vi "Default Settings.vi"(8 "error in (no error)":errorcluster, 11 "6 inch CAD Dispense in":refnum<class "6 inch CAD Dispense.lvclass">) -> (0 "error out":errorcluster, 3 "6 inch CAD Dispense out":refnum<class "6 inch CAD Dispense.lvclass">)   [LabVIEW 2020, in "6 inch CAD Dispense.lvclass"]
uses:
  6 inch CAD Dispense.lvclass
  Dispense.lvclass
  CAD Dispense.lvclass
  C:/Users/hep/Documents/CMU gantry/Classes/Routine/Dispense/CAD Dispense/CAD Dispense.lvclass
  C:/Users/hep/Documents/CMU gantry/Classes/Routine/Dispense/CAD Dispense/6 inch CAD Dispense.lvclass
  C:/Users/hep/Documents/CMU gantry/Classes/Routine/Routine.lvclass
  C:/Program Files/National Instruments/LabVIEW 2020/vi.lib/ActorFramework/Actor/Actor.lvclass
  C:/Users/hep/Documents/CMU gantry/Classes/Routine/Dispense/Dispense.lvclass
panel:
  # "This Routine does not Accept Settings"
  # "This Routine Does not Accept Settings"
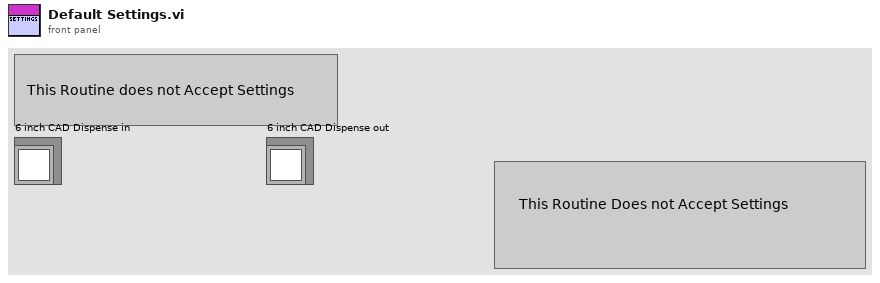
[diagram p1: front panel]
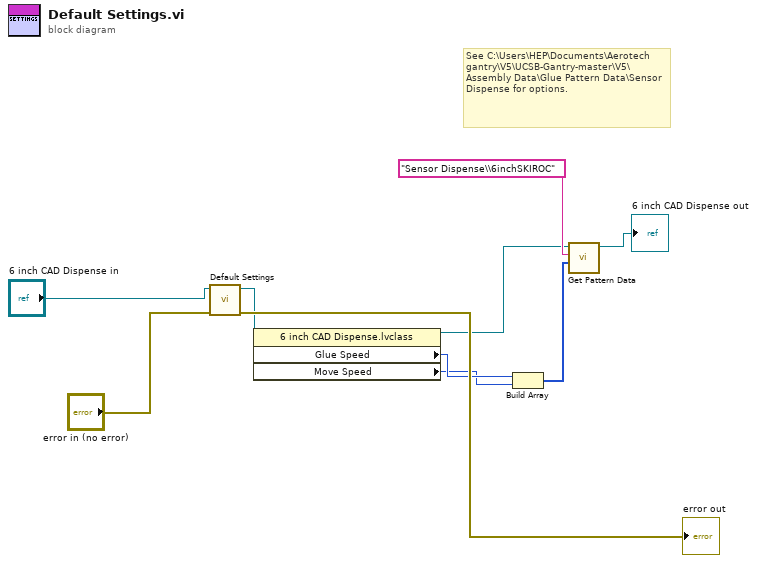
[diagram p0: block diagram]
diagram:
  # "See C:\\Users\\HEP\\Documents\\Aerotech gantry\\V5\\UCSB-Gantry-master\\V5\\Assembly Data\\Glue Pattern Data\\Sensor Dispense for options."
  n1 = call-parent "Default Settings.vi"("error in (no error)"="error in (no error)", "CAD Dispense in"="6 inch CAD Dispense in") -> ("error out"=→"error out":errorcluster, "CAD Dispense out"=w7:refnum<class "6 inch CAD Dispense.lvclass">)  [unwired: 8 in]
  n2 = property class="6 inch CAD Dispense.lvclass"(reference=w7) -> (reference out=w1:refnum<class "6 inch CAD Dispense.lvclass">, "Glue Speed"=w6:i32, "Move Speed"=w5:i32)  [unwired: 1 in, 1 out]
  n3 = Build Array "Build Array"(w6, w5) -> (w4:i32[])
  n4 = call "Get Pattern Data.vi"("File Name"=w4, "Folder Name"="Sensor Dispense\\6inchSKIROC", "Dispense.lvclass"=w1) -> ("Dispense Out"=→"6 inch CAD Dispense out":refnum<class "Dispense.lvclass">)  [unwired: 8 in]
